vi "CvrtCell2Data.vi"(8 "error in (no error)":errorcluster, 9 "ge_HdrNames":T1, 10 "Item Name":string, 11 "Thermocouple in":refnum<class "Thermocouple.lvclass">) -> (0 "error out":errorcluster, 3 "Thermocouple out":refnum<class "Thermocouple.lvclass">)   [LabVIEW 2018, in "Measurement Channels.lvlib" / "Thermocouple.lvclass"]
uses:
  Thermocouple.lvclass
  C:/Users/Jeff Tipps/Documents/DAQMan/source/Classes/Measurements/Class Channel/Channel.lvclass
  Common/Controls/HeaderNames.ctl
  SubVIs Table/Custom Ctls Table/ge_ColType.ctl
  Thermocouple.lvclass/Thermocouple.ctl
  Class Channel/Write Unit_EU.vi
  Class Channel/Channel.lvclass
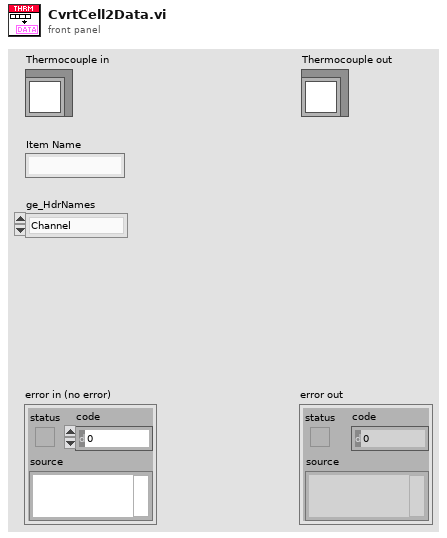
[diagram p1: front panel]
types:
  T1 = typedef "HeaderNames.ctl" = enum16{"Channel", "Device", "Spacer", "Description", "MB", "Range", "Terminal", "Coupling", "Thresh (V)", "Pulse/Rev", "Slope", "Min EU", "Min RPM", "mV/EU", "Iex", "Temp Units", "Type", "CJC Src", "CJC Val", "Ro", "Wire Cfg", "Strain Mode", "Vex", "Bridge Type", "GF", "Gauge Res", "Poisson", "Lead Res", "Init Strain", "GAF", "Scale", "Offset", "Unit (EU)", "dB?", "dB Ref", "Cal Mag", "Cal Units", "Max Temp", "Min Temp", "Max Strain", "Min Strain"}
  T2 = typedef "ge_ColType.ctl" = enum16{"Volts", "Amps", "Ohms", "TermCfg", "WireCfg", "Coup", "Slope", "Iex", "CalUnits", "ThrmUnits", "ThrmType", "CJCSrc", "BrdgType", "Strn Mode", "RTDType"}
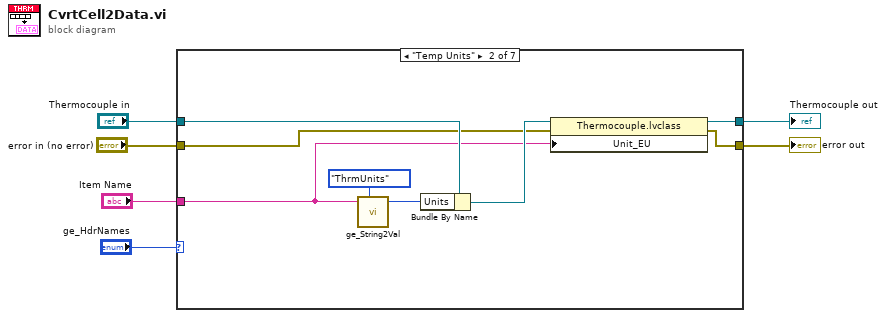
[diagram p0: block diagram]
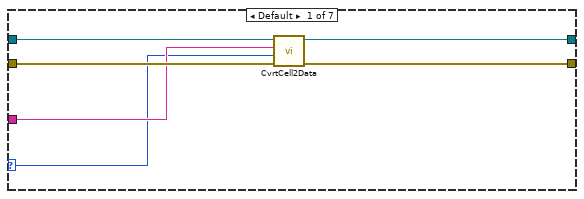
[diagram p2: hidden frame]
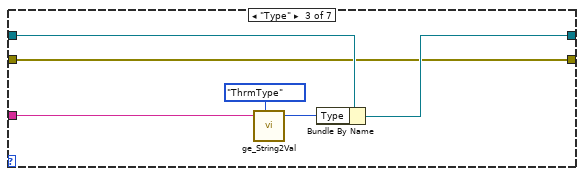
[diagram p3: hidden frame]
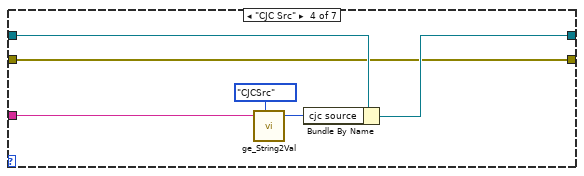
[diagram p4: hidden frame]
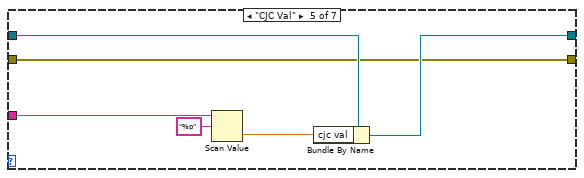
[diagram p5: hidden frame]
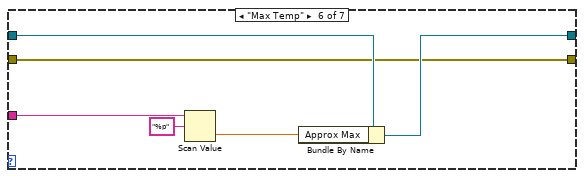
[diagram p6: hidden frame]
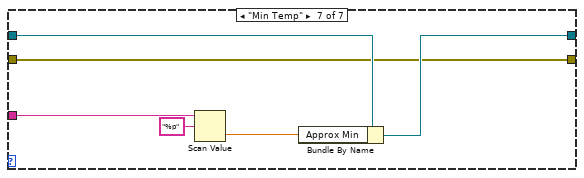
[diagram p7: hidden frame]
diagram:
  n1 = case shown="\"Temp Units\"" "ge_HdrNames" {
    selector: "ge_HdrNames" -> [w7 _ _ _ _ _ _]
    tunnel: "error in (no error)" -> [w12 w14 w21 w27 w36 w42 w48]
    tunnel: [w11 w15 w21 w27 w36 w42 w48] -> w5
    tunnel: [w10 w16 w25 w31 w37 w43 w49] -> w4
    tunnel: "Item Name" -> [w8 w13 w22 w28 w34 w39 w46]
    tunnel: "Thermocouple in" -> [w9 w20 w26 w32 w38 w44 w50]
    frame Default {
      n2 = call-parent "CvrtCell2Data.vi"("error in (no error)"=w12, "Header Names"=w7, "Item Name"=w8, "Channel in"=w9) -> ("error out"=w11:errorcluster, "Channel out"=w10:refnum<class "Thermocouple.lvclass">)  [unwired: 6 in]
    }
    frame "Temp Units" {
      n3 = call "ge_String2Val.vi"("String"=w13, "ColType"=ge_ColType."ThrmUnits") -> ("Value"=w18:u16)  [unwired: 4 in, 1 out]
      n4 = Bundle By Name(cluster=w20, "Units"=w18) -> (w17:refnum<class "Thermocouple.lvclass">)
      n5 = property class="Thermocouple.lvclass"(reference=w17, error in=w14, "Unit_EU"=w13) -> (reference out=w16:refnum<class "Thermocouple.lvclass">, error out=w15:errorcluster)
    }
    frame "Type" {
      n6 = call "ge_String2Val.vi"("String"=w22, "ColType"=ge_ColType."ThrmType") -> ("Value"=w23:u16)  [unwired: 4 in, 1 out]
      n7 = Bundle By Name(cluster=w26, "Type"=w23) -> (w25:refnum<class "Thermocouple.lvclass">)
    }
    frame "CJC Src" {
      n8 = call "ge_String2Val.vi"("String"=w28, "ColType"=ge_ColType."CJCSrc") -> ("Value"=w29:u16)  [unwired: 4 in, 1 out]
      n9 = Bundle By Name(cluster=w32, "cjc source"=w29) -> (w31:refnum<class "Thermocouple.lvclass">)
    }
    frame "CJC Val" {
      n10 = Scan Value(string=w34, format string="%p") -> (value=w33:dbl)  [unwired: 1 in, 1 out]
      n11 = Bundle By Name(cluster=w38, "cjc val"=w33) -> (w37:refnum<class "Thermocouple.lvclass">)
    }
    frame "Max Temp" {
      n12 = Scan Value(string=w39, format string="%p") -> (value=w40:dbl)  [unwired: 1 in, 1 out]
      n13 = Bundle By Name(cluster=w44, "Approx Max"=w40) -> (w43:refnum<class "Thermocouple.lvclass">)
    }
    frame "Min Temp" {
      n14 = Scan Value(string=w46, format string="%p") -> (value=w45:dbl)  [unwired: 1 in, 1 out]
      n15 = Bundle By Name(cluster=w50, "Approx Min"=w45) -> (w49:refnum<class "Thermocouple.lvclass">)
    }
  }
  "error out" <- w5
  "Thermocouple out" <- w4
